vi "Read Process Variables.vi"(0 "VISA resource name":refnum<visa-resource-name>, 1 "Unit Address (1)":u8=1 min=1 max=254, 11 "error in (no error)":errorcluster) -> (4 "VISA resource name out":refnum<visa-resource-name>, 6 "Process Value":sgl, 10 "Measured Value":sgl, 15 "error out":errorcluster)   [LabVIEW 2010, in "Eurotherm 32xx Series.lvlib"]
doc: "This VI returns Process Value and associated variable."
uses:
  <instrlib>/Eurotherm 32xx Series/Eurotherm 32xx Series.lvlib
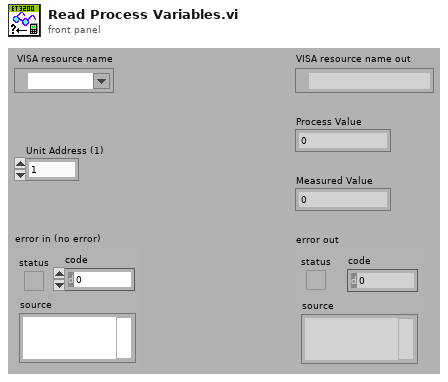
[diagram p1: front panel]
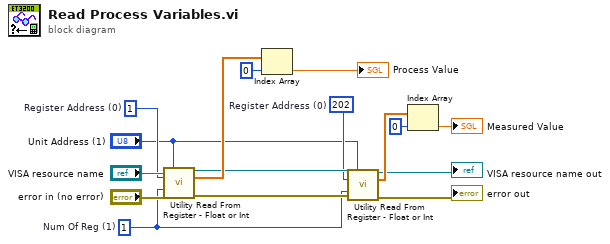
[diagram p0: block diagram]
diagram:
  w9 = u16 202  # Register Address (0)
  w14 = u16 1  # Register Address (0)
  w1 = u16 1  # Num Of Reg (1)
  n1 = call <instrlib>:"Utility Read From Register - Float or Int.vi"("VISA resource name"="VISA resource name", "Unit Address (1)"="Unit Address (1)", "Register Address (0)"=w14, "Num Of Reg (1)"=w1, "error in (no error)"="error in (no error)") -> ("VISA resource name out"=w10:refnum<visa-resource-name>, "Data"=w13:sgl[], "error out"=w11:errorcluster)  [unwired: 8 in]
  n2 = Index Array(array=w13, index=0) -> (element=→"Process Value":sgl)
  n3 = call <instrlib>:"Utility Read From Register - Float or Int.vi"("VISA resource name"=w10, "Unit Address (1)"="Unit Address (1)", "Register Address (0)"=w9, "Num Of Reg (1)"=w1, "error in (no error)"=w11) -> ("VISA resource name out"=→"VISA resource name out":refnum<visa-resource-name>, "Data"=w7:sgl[], "error out"=→"error out":errorcluster)  [unwired: 8 in]
  n4 = Index Array(array=w7, index=0) -> (element=→"Measured Value":sgl)
